vi "DAQmx Find Existing Task.vi"(8 "error in (no error)":errorcluster, 9 "Channels":tag, 11 "Tasks in":refnum<k21>[](array[refnum])) -> (0 "error out":errorcluster, 1 "Task out":refnum<k21>, 2 "Task Index":i32, 3 "Tasks out":refnum<k21>[](array[refnum]))   [LabVIEW 2019, in "DAQmx.lvclass"]
uses:
  DAQmx.lvclass
  <resource>/objmgr/daqmx.rc
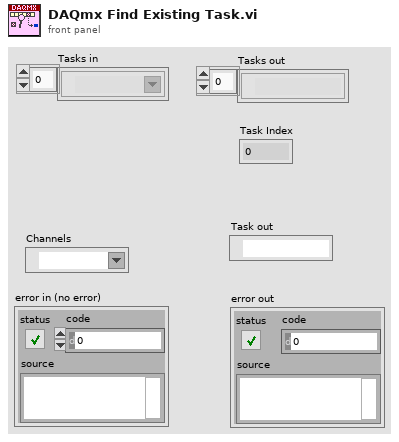
[diagram p1: front panel]
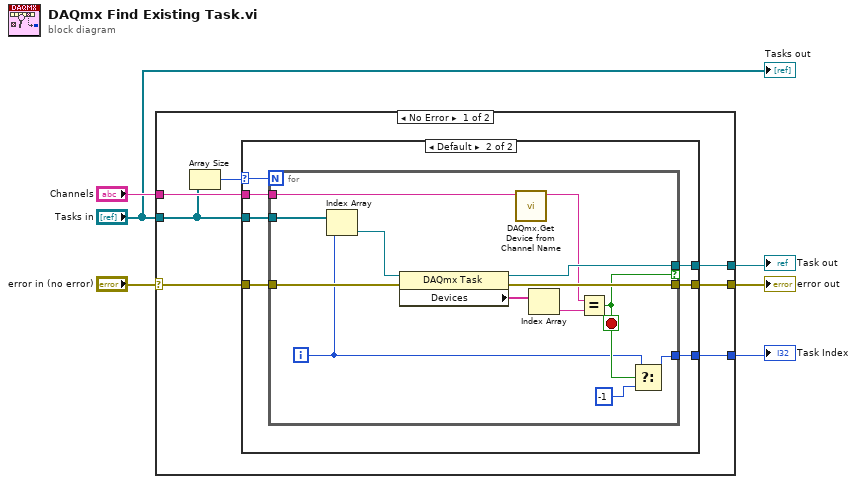
[diagram p0: block diagram]
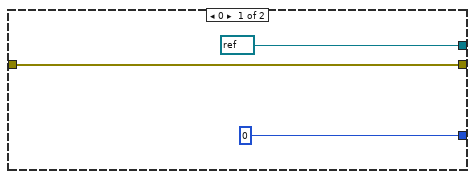
[diagram p2: hidden frame]
diagram:
  n1 = case shown="No Error" "error in (no error)" {
    selector: "error in (no error)" -> [w11 w37]
    tunnel: "Tasks in" -> [w7 _]
    tunnel: "Channels" -> [w12 _]
    tunnel: [w10 w37] -> w4
    tunnel: [w9 _] -> w3
    tunnel: [w8 _] -> w2
    frame No Error {
      n2 = Array Size(array=w7) -> (size(s)=w13:i32)
      n3 = case shown="Default" w13 {
        selector: w13 -> [_ w21]
        tunnel: w12 -> [_ w23]
        tunnel: [refnum<k21> refnum ("Refnum out") w22] -> w9
        tunnel: w7 -> [_ w20]
        tunnel: [0 w19] -> w8
        tunnel: w11 -> [w14 w18]
        tunnel: [w14 w17] -> w10
        frame 0 {
        }
        frame Default {
          n4 = for {
            N: w21 -> [_]
            tunnel: w20 -> [w33]
            tunnel: w23 -> [w25]
            tunnel: [w34] -> w22 if=w29
            tunnel: [w26] -> w19
            tunnel: w18 -> [w32]
            tunnel: [w31] -> w17
            i -> [w27]
            stop <- w29 stop-if-true
            n5 = Index Array(array=w33, index=w27) -> (element=w30:refnum<k21>)
            n6 = property class="DAQmx Task"(reference=w30, error in=w32) -> (reference out=w34:refnum<k21>, error out=w31:errorcluster, "Devices"=w36:tag[])
            n7 = call "DAQmx.Get Device from Channel Name.vi"("Channel"=w25) -> ("Device"=w24:tag)  [unwired: 10 in]
            n8 = Index Array(array=w36) -> (element=w35:tag)  [unwired: 1 in]
            n9 = Equal?(x=w24, y=w35) -> (x = y?=w29:bool)
            n10 = Select(t=w27, s=w29, f=-1) -> (s? t:f=w26:i32)
          }
        }
      }
    }
    frame Error {
    }
  }
  "error out" <- w4
  "Task Index" <- w2
  "Task out" <- w3
  "Tasks out" <- "Tasks in"
